vi "SearchFolders.vi"(8 "error in":errorcluster, 10 "regular expression":string="SwtX", 11 "file path":path=path "D:/Minecraft/mmc-stable-win32/MultiMC/instances/TRAINS 3-/.minecraft/saves/trains/opencomputers/442cd0d6-e139-46e7-881b-600456d36bc7/home") -> (0 "error out":errorcluster, 2 "String Array":string[](array[string]), 3 "Path Array":path[](array[path]), 5 "Root Path Array":path[](array[path]))   [LabVIEW 2014]
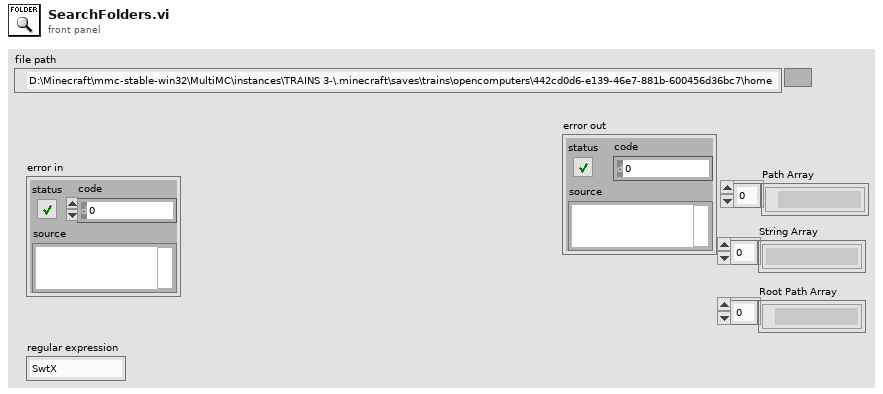
[diagram p1: front panel]
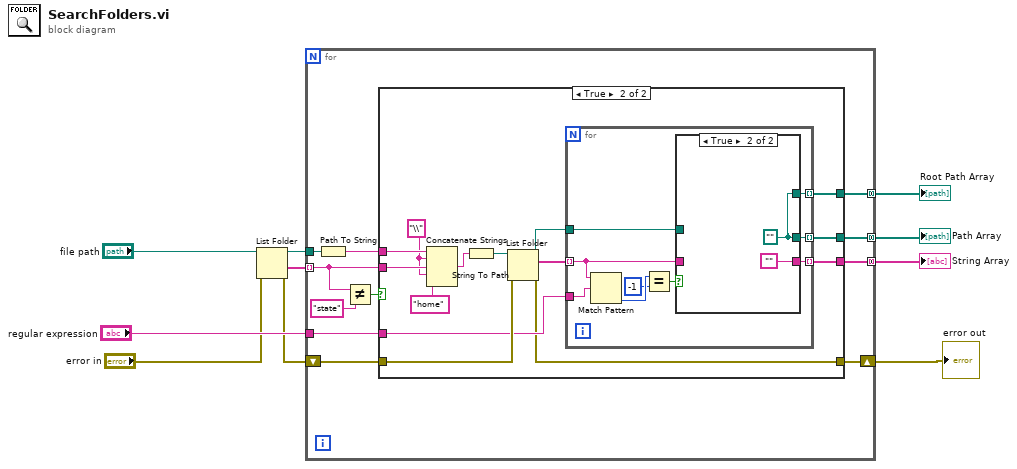
[diagram p0: block diagram]
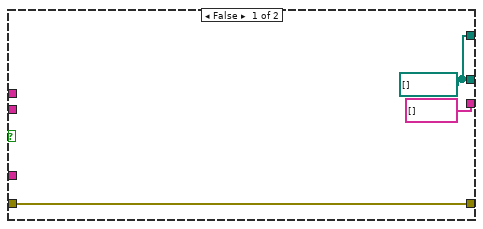
[diagram p2: hidden frame]
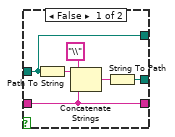
[diagram p3: hidden frame]
diagram:
  n1 = List Folder(path="file path", error in="error in") -> (path out=w3:path, folder names=w4:string[], error out=w2:errorcluster)  [unwired: 2 in, 1 out]
  n2 = for {
    tunnel: w4 -> [w19] mode=indexing
    tunnel: w3 -> [w18]
    tunnel: [w16] -> w6 mode=concatenating
    tunnel: [w15] -> w5 mode=concatenating
    tunnel: "regular expression" -> [w14]
    shift-right: [w13] -> w8
    shift-left: w2 -> [w12]
    tunnel: [w11] -> w1 mode=concatenating
    n3 = Path To String(path=w18) -> (string=w17:string)
    n4 = Not Equal?(x=w19, y="state") -> (x != y?=w20:bool)
    n5 = case shown="True" w20 {
      tunnel: w19 -> [_ w37]
      tunnel: w17 -> [_ w38]
      tunnel: [string[] [] w33] -> w16
      tunnel: [w22 w31] -> w15
      tunnel: w12 -> [w23 w30]
      tunnel: w14 -> [_ w29]
      tunnel: [w23 w28] -> w13
      tunnel: [w22 w27] -> w11
      frame False {
        w22 = path[] []
      }
      frame True {
        w26 = "\\" ("string")
        n6 = Concatenate Strings(w38, w26, w37, w26, "home" ("string")) -> (w36:string)
        n7 = String To Path(string=w36) -> (path=w35:path)
        n8 = List Folder(path=w35, error in=w30) -> (path out=w32:path, filenames=w34:string[], error out=w28:errorcluster)  [unwired: 2 in, 1 out]
        n9 = for {
          tunnel: w34 -> [w42] mode=indexing
          tunnel: [w41] -> w33 mode=indexing
          tunnel: w32 -> [w47]
          tunnel: [w46] -> w31 mode=indexing
          tunnel: w29 -> [w43]
          tunnel: [w39] -> w27 mode=indexing
          n10 = Match Pattern(string=w42, regular expression=w43) -> (offset past match=w45:i32)  [unwired: 1 in, 3 out]
          n11 = Equal?(x=w45, y=-1) -> (x = y?=w40:bool)
          n12 = case shown="True" w40 {
            tunnel: w47 -> [w48 _]
            tunnel: [w50 w54] -> w46
            tunnel: w42 -> [w49 _]
            tunnel: [w49 ""] -> w41
            tunnel: [w48 w54] -> w39
            frame False {
              n13 = Path To String(path=w48) -> (string=w52:string)
              n14 = Concatenate Strings(w52, "\\" ("string"), w49) -> (w51:string)
              n15 = String To Path(string=w51) -> (path=w50:path)
            }
            frame True {
              w54 = path ""
            }
          }
        }
      }
    }
  }
  "error out" <- w8
  "String Array" <- w6
  "Path Array" <- w5
  "Root Path Array" <- w1
